vi "ULx_Functions.vi"() -> ()   [LabVIEW 2017]
uses:
  <vilib>/ULx/Create Channel.llb/ULx Create Channel (AI-Voltage-Basic).vi
  <vilib>/ULx/Timing.llb/ULx Timing (Sample Clock).vi
  <vilib>/ULx/Read.llb/ULx Read (Analog Wfm 1Chan 1Samp).vi
panel:
  in  "physical channels":refnum<k21>
  out "Waveform Graph":waveform(dbl)(graph)
  in  "rate":dbl=1000.0
  in  "samples per channel":i32=1000
  in  "sample mode":i32(ring) items=["FiniteSamples", "ContinuousSamples"]
  in  "minimum value":dbl=-5.0
  in  "maximum value":dbl=5.0
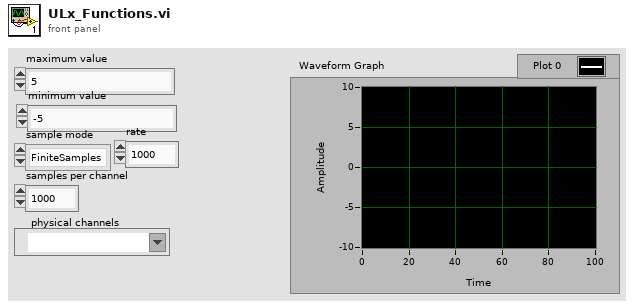
[diagram p1: front panel]
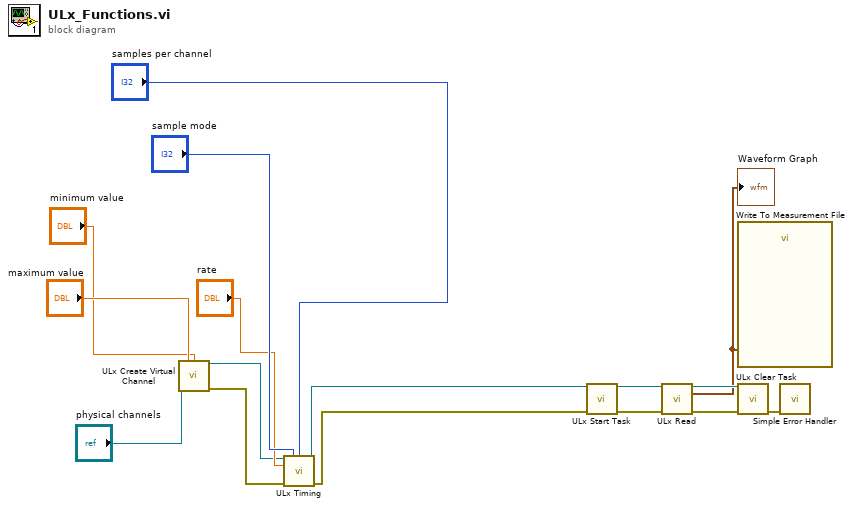
[diagram p0: block diagram]
diagram:
  n1 = call-poly <vilib>:"ULx Create Virtual Channel.vi"("maximum value"="maximum value", "minimum value"="minimum value", "physical channels"="physical channels") -> ("task out"=w3:refnum<k24>, "error out"=w2:errorcluster)  [unwired: 11 in]
  n2 = call-poly <vilib>:"ULx Timing.vi"("task in"=w3, "sample mode"="sample mode", "samples per channel"="samples per channel", "rate"="rate", "error in"=w2) -> ("task out"=w4:refnum<k24>, "error out"=w5:errorcluster)  [unwired: 9 in]
  n3 = call <vilib>:"ULx Start Task.vi"("task in"=w4, "error in"=w5) -> ("task out"=w13:refnum<k24>, "error out"=w12:errorcluster)  [unwired: 12 in]
  n4 = call-poly <vilib>:"ULx Read.vi"("task in"=w13, "error in"=w12) -> ("task out"=w11:refnum<k24>, "data"=w9:waveform(dbl), "error out"=w10:errorcluster)  [unwired: 11 in]
  "Waveform Graph" <- w9
  n5 = call "Write To Measurement File"("Signals"=w9) -> ()  [unwired: 16 in, 3 out]
  n6 = call <vilib>:"ULx Clear Task.vi"("task in"=w11, "error in"=w10) -> ("error out"=w14:errorcluster)  [unwired: 13 in]
  n7 = call <vilib>:"Simple Error Handler.vi"("error in (no error)"=w14) -> ()  [unwired: 4 in, 5 out]
